vi "IntegerAsValue.vi"(8 "error in":errorcluster, 11 "scalar value (int32)":i32) -> (0 "error out":errorcluster, 3 "scalar string":string)   [LabVIEW 2014]
doc: "Format a LV integer (I32) as an XML-RPC integer"
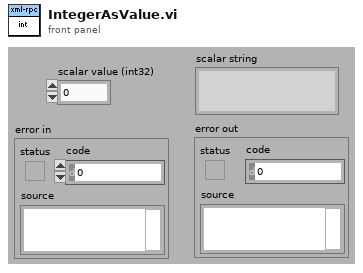
[diagram p1: front panel]
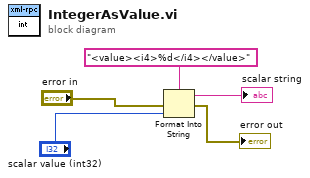
[diagram p0: block diagram]
diagram:
  n1 = Format Into String(format string="<value><i4>%d</i4></value>", error in="error in", "scalar value (int32)") -> (resulting string=→"scalar string":string, error out=→"error out":errorcluster)  [unwired: 1 in]
